vi "H5Ocopy.vi"(4 "lcpl_id":T1, 6 "ocpypl_id":T1, 7 "Source Name":string=".", 8 "error in (no error)":errorcluster, 9 "Source Location Ref":T1, 10 "Destination Name":string, 11 "Dest Location Ref":T1) -> (0 "error out":errorcluster, 1 "Source Location Ref out":T1, 3 "Dest Location Ref out":T1)   [LabVIEW 2017]
doc: "Copies an object in an HDF5 file."
uses:
  <vilib>/UPVI/lvhdf5/library.llb/HDF5 Ref.ctl
  <vilib>/UPVI/lvhdf5/hdf5.dll
panel:
  # "LVHDF5 Toolkit\nCopyright (c) 2005-2013 by Jason D. Sommerville\nCopyright (c) 2014-2015 by UPVI, LLC.\n\nThis use and distribution of this file is governed by the terms found in \nLICENSE.txt distributed with this toolkit and installed at\n <user.lib>\\_lvhdf5\\LICENSE.txt"
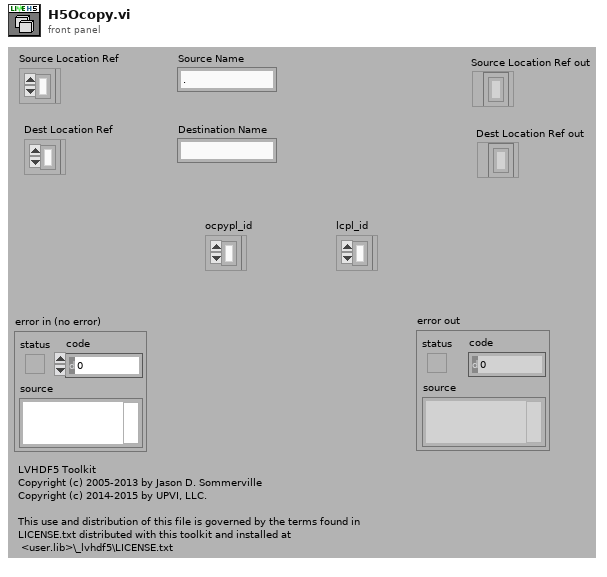
[diagram p1: front panel]
types:
  T1 = typedef "HDF5 Ref.ctl" = refnum<k1>
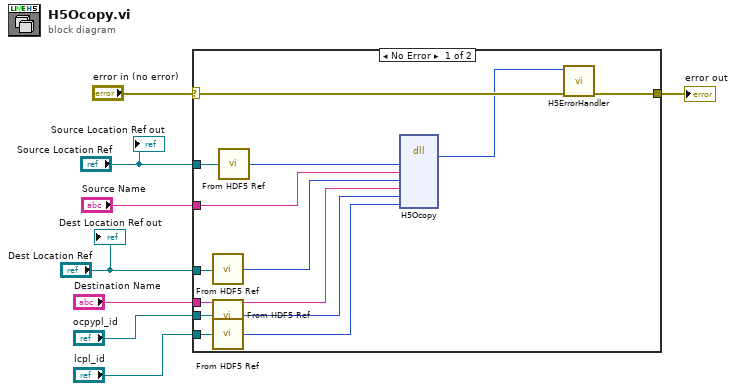
[diagram p0: block diagram]
diagram:
  n1 = case shown="No Error" "error in (no error)" {
    selector: "error in (no error)" -> [w21 w22]
    tunnel: [w20 w22] -> w7
    tunnel: "Source Location Ref" -> [w19 _]
    tunnel: "Source Name" -> [w13 _]
    tunnel: "lcpl_id" -> [w18 _]
    tunnel: "Dest Location Ref" -> [w14 _]
    tunnel: "Destination Name" -> [w11 _]
    tunnel: "ocpypl_id" -> [w10 _]
    frame No Error {
      n2 = call <vilib>:"From HDF5 Ref.vi"("HDF5 Ref"=w14) -> ("I32"=w12:i32)
      n3 = call <vilib>:"From HDF5 Ref.vi"("HDF5 Ref"=w10) -> ("I32"=w9:i32)
      n4 = call <vilib>:"From HDF5 Ref.vi"("HDF5 Ref"=w18) -> ("I32"=w17:i32)
      n5 = call <vilib>:"From HDF5 Ref.vi"("HDF5 Ref"=w19) -> ("I32"=w16:i32)
      n6 = dll-call lib="C:/Program Files/National Instruments/LabVIEW 2017/vi.lib/UPVI/lvhdf5/hdf5.dll" fn="H5Ocopy"("src_loc_id"=w16, "src_name"=w13, "dest_loc_id"=w12, "dest_name"=w11, "lcpl_id"=w9, "lapl_id"=w17) -> ("return type"=w15:i32)  [unwired: 9 in, 2 out]
      n7 = call <vilib>:"H5ErrorHandler.vi"("error in (no error)"=w21, "herr_t"=w15) -> ("error out"=w20:errorcluster)  [unwired: 3 in, 4 out]
    }
    frame Error {
    }
  }
  "error out" <- w7
  "Source Location Ref out" <- "Source Location Ref"
  "Dest Location Ref out" <- "Dest Location Ref"
